vi "healthAndStatusTest.vi"() -> ()   [LabVIEW 2016]
uses:
  Common_FPGA_HealthAndStatus/DataTypes/HealthAndStatusSettings.ctl
  Common_FPGA_HealthAndStatus/DataTypes/HealthAndStatusUpdateMode.ctl
  <vilib>/rvi/Emulation/niFpgaGetClockAttributes.vi
  <vilib>/rvi/Emulation/niFpgaSctlEmulationGetInTimedLoop.vi
  <vilib>/rvi/Emulation/niFpgaEmulationReportErrorSimple.vi
  <vilib>/rvi/eio/common/nirviEmuTemplateMethod_errors.vi
  <vilib>/rvi/Emulation/niFpgaCriticalErrorInLSC.vi
  <vilib>/rvi/Emulation/niFpgaProcessEmulError.vi
  <vilib>/eio/EIOMethodNode/EIOMethodNode.xnode
  Common_FPGA_HealthAndStatus/FPGAHealthAndStatus.lvlib
panel:
  in  "Bit":i16
  in  "SetBit":bool
  in  "Clear":bool
  in  "Sub0":bool
  in  "Add0":bool
  in  "Set0":bool
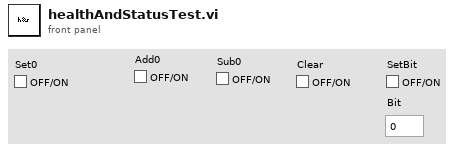
[diagram p1: front panel]
types:
  T1 = typedef "FPGAHealthAndStatus.lvlib/HealthAndStatusSettings.ctl" = cluster{"InternalHealthAndStatusFIFO":refnum<k21>, "HealthAndStatusQueryFIFO":refnum<k21>, "HealthAndStatusResponseFIFO":refnum<k21>, "HealthAndStatusMemory":refnum<k21>, "MemorySize":i32}
  T2 = typedef "FPGAHealthAndStatus.lvlib/HealthAndStatusUpdateMode.ctl" = enum8{"NOP", "Set", "Add", "Subtract", "Or"}
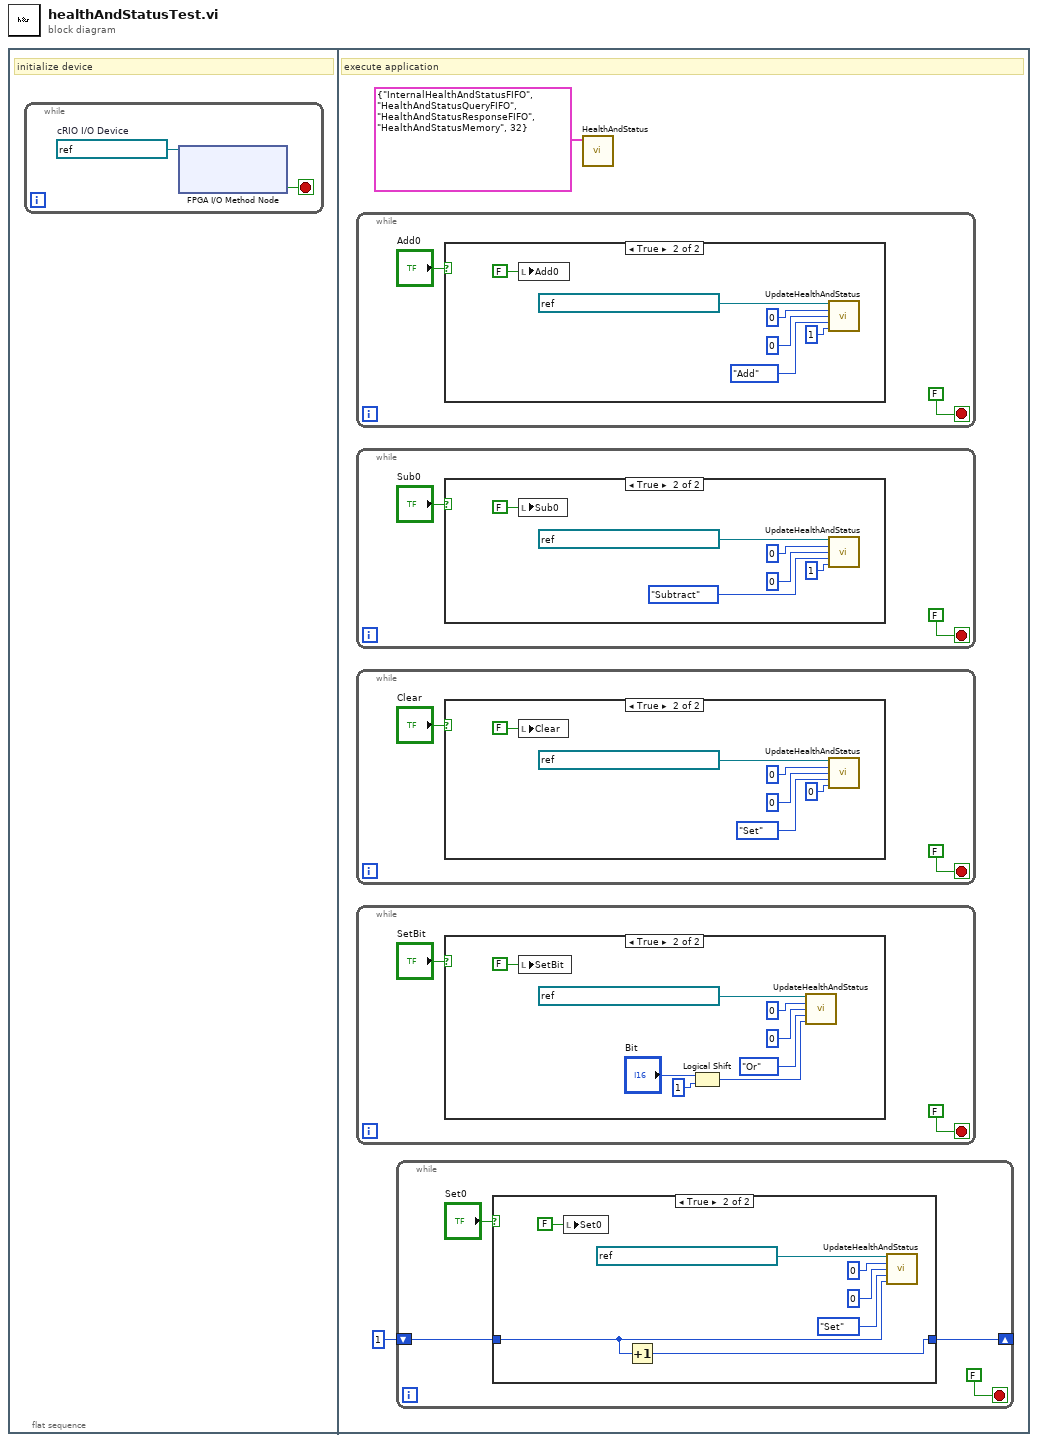
[diagram p0: block diagram]
diagram:
  n1 = flat-sequence {
    frame #0 {
      # "initialize device"
      n2 = while {
        stop <- w1 stop-if-true
        w2 = refnum<k21> "ModbusPort1-4"  # cRIO I/O Device
        n3 = xnode "FPGA I/O Method Node"("FPGA I/O In"=w2) -> ("Ready"=w1:bool)  [unwired: 1 out]
      }
    }
    frame #1 {
      # "execute application"
      n4 = while {
        stop <- FALSE stop-if-true
        n5 = case shown="True" "Add0" {
          frame False {
          }
          frame True {
            n6 = local write "Add0"(FALSE ("OrBit3")) -> ()
            n7 = call "UpdateHealthAndStatus.vi"("InternalHealthAndStatusFIFO"=refnum<k21> "InternalHealthAndStatusFIFO", "AddressOffset"=u32 0, "BaseAddress"=u32 0, "HealthAndStatusUpdateMode"=HealthAndStatusUpdateMode."Add", "Data"=u32 1) -> ()  [unwired: 11 in]
          }
        }
      }
      n8 = while {
        stop <- FALSE stop-if-true
        n9 = case shown="True" "Sub0" {
          frame False {
          }
          frame True {
            n10 = local write "Sub0"(FALSE ("OrBit3")) -> ()
            n11 = call "UpdateHealthAndStatus.vi"("InternalHealthAndStatusFIFO"=refnum<k21> "InternalHealthAndStatusFIFO", "AddressOffset"=u32 0, "BaseAddress"=u32 0, "HealthAndStatusUpdateMode"=HealthAndStatusUpdateMode."Subtract", "Data"=u32 1) -> ()  [unwired: 11 in]
          }
        }
      }
      n12 = while {
        stop <- FALSE stop-if-true
        n13 = case shown="True" "Clear" {
          frame False {
          }
          frame True {
            n14 = local write "Clear"(FALSE ("OrBit3")) -> ()
            n15 = call "UpdateHealthAndStatus.vi"("InternalHealthAndStatusFIFO"=refnum<k21> "InternalHealthAndStatusFIFO", "AddressOffset"=u32 0, "BaseAddress"=u32 0, "HealthAndStatusUpdateMode"=HealthAndStatusUpdateMode."Set", "Data"=u32 0) -> ()  [unwired: 11 in]
          }
        }
      }
      n16 = while {
        stop <- FALSE stop-if-true
        n17 = case shown="True" "SetBit" {
          frame False {
          }
          frame True {
            n18 = local write "SetBit"(FALSE ("OrBit3")) -> ()
            n19 = Logical Shift(y="Bit", x=i16 1) -> (x << y=w7:i16)
            n20 = call "UpdateHealthAndStatus.vi"("InternalHealthAndStatusFIFO"=refnum<k21> "InternalHealthAndStatusFIFO", "AddressOffset"=u32 0, "BaseAddress"=u32 0, "HealthAndStatusUpdateMode"=HealthAndStatusUpdateMode."Or", "Data"=w7) -> ()  [unwired: 11 in]
          }
        }
      }
      n21 = while {
        shift-right: [w39] -> _
        shift-left: i16 1 -> [w40]
        stop <- FALSE stop-if-true
        n22 = case shown="True" "Set0" {
          tunnel: w40 -> [w43 w44]
          tunnel: [w43 w45] -> w39
          frame False {
          }
          frame True {
            n23 = local write "Set0"(FALSE ("OrBit3")) -> ()
            n24 = Increment(x=w44) -> (x+1=w45:i16)
            n25 = call "UpdateHealthAndStatus.vi"("InternalHealthAndStatusFIFO"=refnum<k21> "InternalHealthAndStatusFIFO", "AddressOffset"=u32 0, "BaseAddress"=u32 0, "HealthAndStatusUpdateMode"=HealthAndStatusUpdateMode."Set", "Data"=w44) -> ()  [unwired: 11 in]
          }
        }
      }
      n26 = call "HealthAndStatus.vi"("HealthAndStatusSettings"=T1 {"InternalHealthAndStatusFIFO"="InternalHealthAndStatusFIFO", "HealthAndStatusQueryFIFO"="HealthAndStatusQueryFIFO", "HealthAndStatusResponseFIFO"="HealthAndStatusResponseFIFO", "HealthAndStatusMemory"="HealthAndStatusMemory", "MemorySize"=32}) -> ()  [unwired: 11 in]
    }
  }
